vi "Global-force-controller-test.vi"() -> ()   [LabVIEW 2020]
uses:
  Global-force.vi
panel:
  in  "stop":bool
  in  "Numeric":dbl
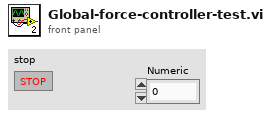
[diagram p1: front panel]
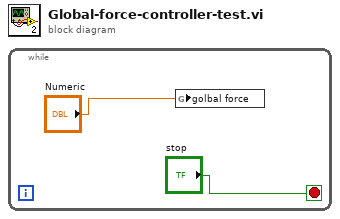
[diagram p0: block diagram]
diagram:
  n1 = while {
    stop <- "stop" stop-if-true
    n2 = global write "Global-force.vi" "golbal force"("Numeric") -> ()
  }
